vi "Normalized CC U16.vi"(0 "Template U16":u16[][](array[numeric]), 7 "A U16":T1, 11 "Error In":errorcluster) -> (4 "normxcorr2":dbl[][](array[numeric]), 8 "Max Value":dbl, 15 "Error Out":errorcluster)   [LabVIEW 2020]
uses:
  <vilib>/vision/Image Controls.llb/IMAQ Image.ctl
  <vilib>/Analysis/2dsp.llb/2D Cross Correlation (CDB).vi
  <vilib>/Analysis/NI_AALPro.lvlib
  <vilib>/Analysis/NI_AALBase.lvlib
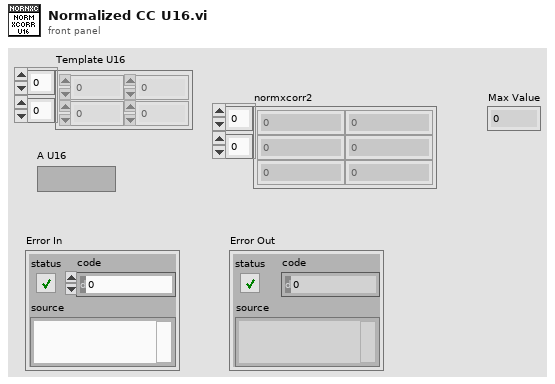
[diagram p1: front panel]
types:
  T1 = typedef "IMAQ Image.ctl" = refnum<image>
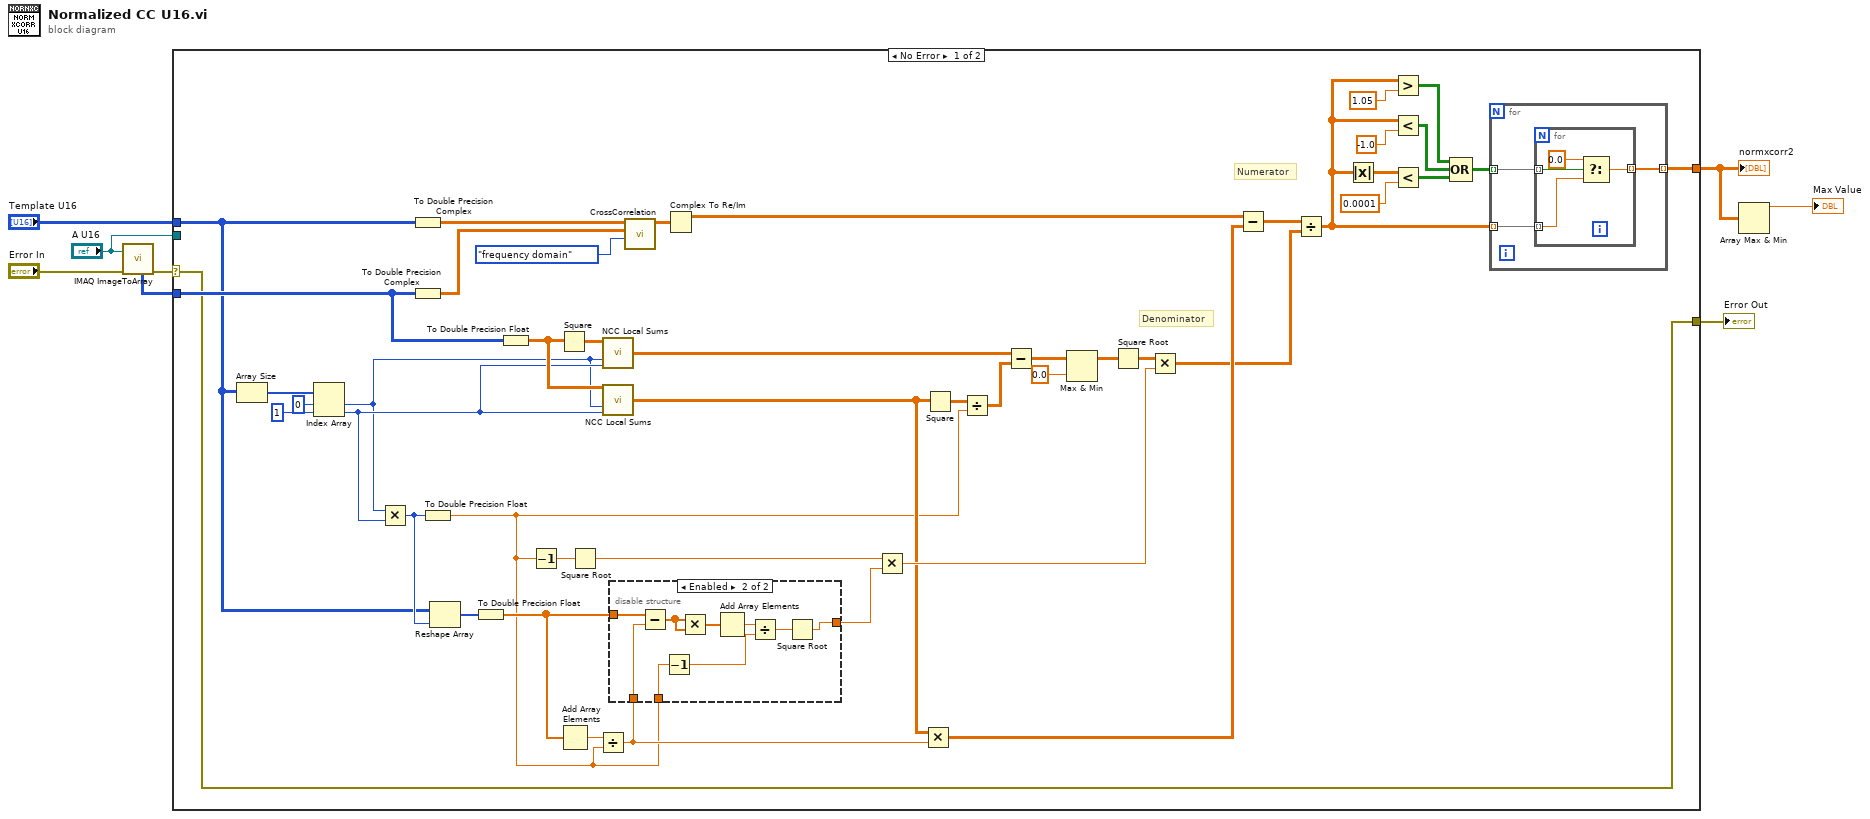
[diagram p0: block diagram]
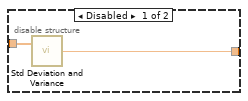
[diagram p2: hidden frame]
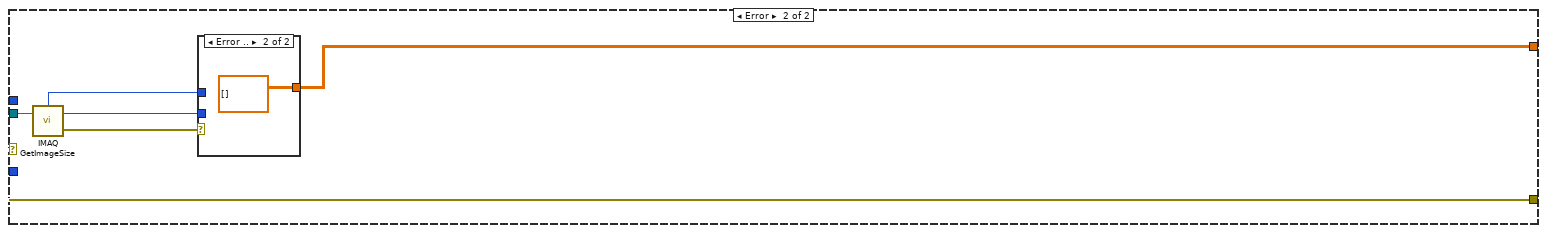
[diagram p3: hidden frame]
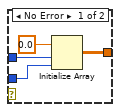
[diagram p4: hidden frame]
diagram:
  n1 = call "IMAQ ImageToArray"("error in (no error)"="Error In", "Image"="A U16") -> ("Image Pixels (U16)"=w8:u16[][], "error out"=w7:errorcluster)  [unwired: 2 in, 3 out]
  n2 = case shown="No Error" w7 {
    selector: w7 -> [w15 w73]
    tunnel: [w24 w75] -> w2
    tunnel: w8 -> [w16 _]
    tunnel: "Template U16" -> [w14 _]
    tunnel: "A U16" -> [_ w78]
    tunnel: [w15 w73] -> w5
    frame No Error {
      # "Denominator"
      # "Numerator"
      n3 = Array Size(array=w14) -> (size(s)=w13:i32[])
      n4 = Index Array(array=w13, index #1=0 ("index"), index #2=1 ("index")) -> (element #1=w9:i32, element #2=w10:i32)
      n5 = Multiply(x=w9, y=w10) -> (x*y=w41:i32)
      n6 = To Double Precision Complex(1:w14) -> (0:w53:cdb[][])
      n7 = To Double Precision Complex(1:w16) -> (0:w52:cdb[][])
      n8 = To Double Precision Float(number=w41) -> (double precision float=w27:dbl)
      n9 = Reshape Array(w14, w41) -> (w40:u16[])
      n10 = To Double Precision Float(number=w40) -> (double precision float=w35:dbl[])
      n11 = To Double Precision Float(number=w16) -> (double precision float=w49:dbl[][])
      n12 = Decrement(x=w27) -> (x-1=w42:dbl)
      n13 = Square(x=w49) -> (x^2=w50:dbl[][])
      n14 = Add Array Elements(numeric array=w35) -> (sum=w34:dbl)
      n15 = Square Root(x=w42) -> (sqrt(x)=w39:dbl)
      n16 = Divide(x=w34, y=w27) -> (x/y=w28:dbl)
      n17 = call "NCC Local Sums.vi"("Input Array"=w50, "Row Pad"=w9, "Col Pad"=w10) -> ("Local Sum"=w48:dbl[][])  [unwired: 12 in]
      n18 = call "NCC Local Sums.vi"("Input Array"=w49, "Row Pad"=w9, "Col Pad"=w10) -> ("Local Sum"=w33:dbl[][])  [unwired: 12 in]
      n19 = disable-structure shown="Enabled" {
        disable-tunnel: w35 -> [w63 w72]
        disable-tunnel: [w62 w64] -> w29
        disable-tunnel: w28 -> [_ w71]
        disable-tunnel: w27 -> [_ w67]
        frame Disabled {
          n20 = call <vilib>:"Std Deviation and Variance.vi"("X"=w63) -> ("standard deviation"=w62:dbl)  [unwired: 1 in, 2 out]
        }
        frame Enabled {
          n21 = Subtract(x=w72, y=w71) -> (x-y=w70:dbl[])
          n22 = Decrement(x=w67) -> (x-1=w66:dbl)
          n23 = Multiply(x=w70, y=w70) -> (x*y=w69:dbl[])
          n24 = Add Array Elements(numeric array=w69) -> (sum=w68:dbl)
          n25 = Divide(x=w68, y=w66) -> (x/y=w65:dbl)
          n26 = Square Root(x=w65) -> (sqrt(x)=w64:dbl)
        }
      }
      n27 = call-poly <vilib>:"CrossCorrelation.vi"("algorithm"=enum32{"direct", "frequency domain"}."frequency domain", "Y"=w52, "X"=w53) -> ("Rxy"=w51:cdb[][])  [unwired: 7 in, 1 out]
      n28 = Complex To Re/Im(x + iy=w51) -> (x=w36:dbl[][])  [unwired: 1 out]
      n29 = Multiply(x=w39, y=w29) -> (x*y=w37:dbl)
      n30 = Multiply(x=w33, y=w28) -> (x*y=w32:dbl[][])
      n31 = Square(x=w33) -> (x^2=w47:dbl[][])
      n32 = Divide(x=w47, y=w27) -> (x/y=w46:dbl[][])
      n33 = Subtract(x=w48, y=w46) -> (x-y=w44:dbl[][])
      n34 = Max & Min(x=w44, y=0.0) -> (max(x,y)=w43:dbl[][])  [unwired: 1 out]
      n35 = Square Root(x=w43) -> (sqrt(x)=w38:dbl[][])
      n36 = Multiply(x=w38, y=w37) -> (x*y=w30:dbl[][])
      n37 = Subtract(x=w36, y=w32) -> (x-y=w31:dbl[][])
      n38 = Divide(x=w31, y=w30) -> (x/y=w22:dbl[][])
      n39 = Absolute Value(x=w22) -> (abs(x)=w26:dbl[][])
      n40 = Greater?(x=w22, y=1.05) -> (0:w18:bool[][])
      n41 = Less?(x=w22, y=-1.0) -> (x < y?=w19:bool[][])
      n42 = Less?(x=w26, y=0.0001) -> (x < y?=w20:bool[][])
      n43 = Compound Arithmetic op=OR(w18, w19, w20) -> (w17:bool[][])
      n44 = for {
        tunnel: w22 -> [w57] mode=indexing
        tunnel: w17 -> [w56] mode=indexing
        tunnel: [w55] -> w24 mode=indexing
        n45 = for {
          tunnel: w57 -> [w60] mode=indexing
          tunnel: w56 -> [w61] mode=indexing
          tunnel: [w58] -> w55 mode=indexing
          n46 = Select(t=0.0, s=w61, f=w60) -> (s? t:f=w58:dbl)
        }
      }
    }
    frame Error {
      n47 = call "IMAQ GetImageSize"("Image"=w78) -> ("Y Resolution"=w77:i32, "X Resolution"=w76:i32, "error out"=w74:errorcluster)  [unwired: 3 in]
      n48 = case shown="Error .." w74 {
        tunnel: w77 -> [w81 _]
        tunnel: w76 -> [w82 _]
        tunnel: [w80 dbl[][] []] -> w75
        frame No Error {
          n49 = Initialize Array(0.0 ("element"), w82, w81) -> (w80:dbl[][])
        }
        frame Error {
        }
      }
    }
  }
  "normxcorr2" <- w2
  "Error Out" <- w5
  n50 = Array Max & Min(array=w2) -> (max value=→"Max Value":dbl)  [unwired: 3 out]
